vi "DAQmx.44xx.Coerce Fs.vi"(8 "error in (no error)":errorcluster, 10 "Fs":dbl, 11 "Refnum in":refnum<k21>) -> (0 "error out":errorcluster, 2 "coerced(Fs)":dbl, 3 "Refnum out":refnum<k21>)   [LabVIEW 2019, in "DAQmx.lvclass"]
uses:
  DAQmx.lvclass
  <resource>/objmgr/daqmx.rc
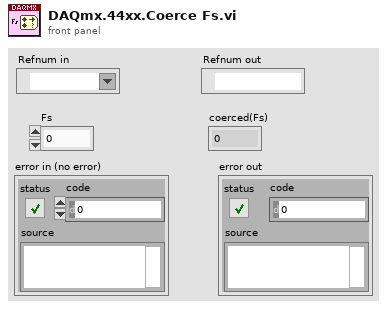
[diagram p1: front panel]
types:
  T1 = typedef "DAQmx.lvclass/DAQ.Config.Device Type--enum.ctl" = enum16{"None", "USB-4431", "PXI-446x"}
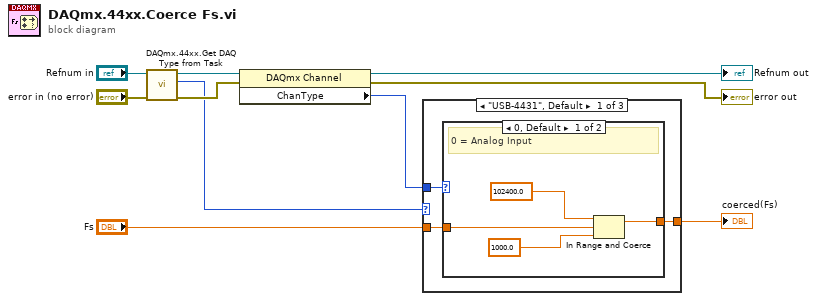
[diagram p0: block diagram]
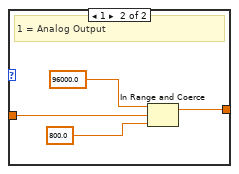
[diagram p2: hidden frame]
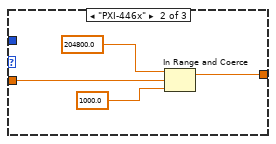
[diagram p3: hidden frame]
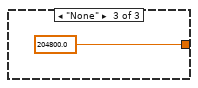
[diagram p4: hidden frame]
diagram:
  n1 = call "DAQmx.44xx.Get DAQ Type from Task.vi"("error in (no error)"="error in (no error)", "Task in"="Refnum in") -> ("error out"=w3:errorcluster, "DAQ Type"=w2:T1, "Task out"=w5:refnum<k21>)  [unwired: 5 in, 2 out]
  n2 = property class="DAQmx Channel"(reference=w5, error in=w3) -> (reference out=→"Refnum out":refnum<k21>, error out=→"error out":errorcluster, "ChanType"=w9:i32)
  n3 = case shown="\"USB-4431\", Default" w2 {
    tunnel: [w13 w22 204800.0 ("upper limit")] -> w7
    tunnel: w9 -> [w12 _ _]
    tunnel: "Fs" -> [w11 w23 _]
    frame "USB-4431", Default {
      n4 = case shown="0, Default" w12 {
        tunnel: [w15 w19] -> w13
        tunnel: w11 -> [w16 w21]
        frame 0, Default {
          # "0 = Analog Input"
          n5 = In Range and Coerce(upper limit=102400.0, x=w16, lower limit=1000.0) -> (coerced(x)=w15:dbl)  [unwired: 1 out]
        }
        frame 1 {
          # "1 = Analog Output"
          n6 = In Range and Coerce(upper limit=96000.0, x=w21, lower limit=800.0) -> (coerced(x)=w19:dbl)  [unwired: 1 out]
        }
      }
    }
    frame "PXI-446x" {
      n7 = In Range and Coerce(upper limit=204800.0, x=w23, lower limit=1000.0) -> (coerced(x)=w22:dbl)  [unwired: 1 out]
    }
    frame "None" {
    }
  }
  "coerced(Fs)" <- w7
